vi "KE622x -- 2182 -A Read.vi"(0 "622x Resource In":refnum<visa-resource-name>, 1 "Check For SCPI Errors? (T)":bool=TRUE, 11 "error in (no error)":errorcluster, 13 "Max Num Bytes To Read (256)":u32=256) -> (4 "622x Resource Out (dupl)":refnum<visa-resource-name>, 8 "2182-A Reponse String":string, 15 "error out":errorcluster)   [LabVIEW 2019, in "Keithley 622x.lvlib"]
uses:
  Keithley 622x.lvlib
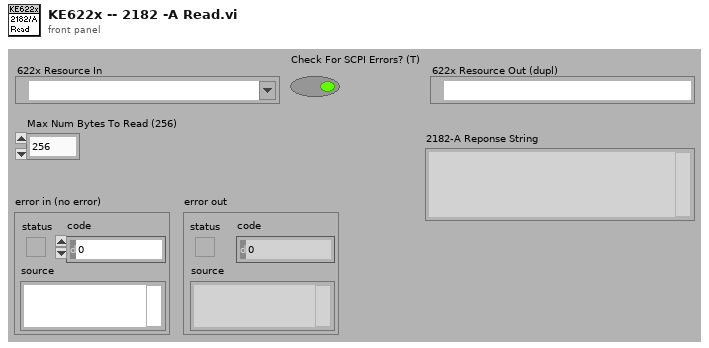
[diagram p1: front panel]
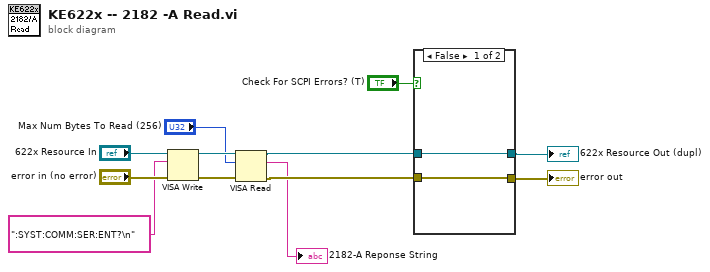
[diagram p0: block diagram]
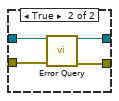
[diagram p2: hidden frame]
diagram:
  n1 = VISA Write(VISA resource name="622x Resource In", write buffer=":SYST:COMM:SER:ENT?\n" ("format string"), error in (no error)="error in (no error)") -> (VISA resource name out=w6:refnum<visa-resource-name>, error out=w5:errorcluster)  [unwired: 1 out]
  n2 = VISA Read(VISA resource name=w6, byte count="Max Num Bytes To Read (256)", error in (no error)=w5) -> (VISA resource name out=w3:refnum<visa-resource-name>, read buffer=→"2182-A Reponse String":string, error out=w2:errorcluster)  [unwired: 1 out]
  n3 = case shown="False" "Check For SCPI Errors? (T)" {
    tunnel: w3 -> [w14 w18]
    tunnel: w2 -> [w13 w17]
    tunnel: [w13 w16] -> w8
    tunnel: [w14 w15] -> w9
    frame False {
    }
    frame True {
      n4 = call "Error Query.vi"("VISA Resource In"=w18, "error in (no error)"=w17) -> ("VISA Resource Out (dupl)"=w15:refnum<visa-resource-name>, "error out"=w16:errorcluster)  [unwired: 10 in, 2 out]
    }
  }
  "622x Resource Out (dupl)" <- w9
  "error out" <- w8
